vi "Get Embedded Message Name.vi"(10 "MessageElementType":T1, 11 "Element Name":string) -> (3 "Embedded Message Name":string)   [LabVIEW 2019, in "grpc-lvsupport.lvlib"]
uses:
  grpc-lvsupport.lvlib
  Message Element Type.ctl
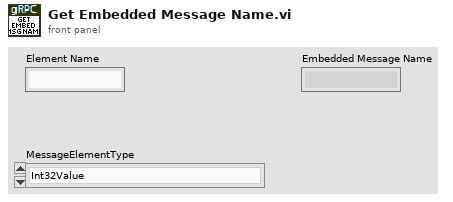
[diagram p1: front panel]
types:
  T1 = typedef "grpc-lvsupport.lvlib/Message Element Type.ctl" = enum32{"Int32Value", "FloatValue", "DoubleValue", "BoolValue", "StringValue", "MessageValue", "Int64Value", "UInt32Value", "UInt64Value", "EnumValue", "Bytes", "Fixed64", "Fixed32", "SFixed64", "SFixed32", "SInt64", "SInt32"}
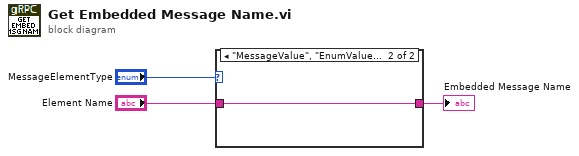
[diagram p0: block diagram]
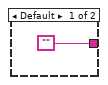
[diagram p2: hidden frame]
diagram:
  n1 = case shown="\"MessageValue\", \"EnumValue\"" "MessageElementType" {
    tunnel: ["" w5] -> w1
    tunnel: "Element Name" -> [_ w5]
    frame Default {
    }
    frame "MessageValue", "EnumValue" {
    }
  }
  "Embedded Message Name" <- w1
